vi "open_MainWindow_dyn.vi"(8 "error in (no error)":errorcluster) -> (0 "error out":errorcluster)   [LabVIEW 2015]
doc: "opens the main window dynamically"
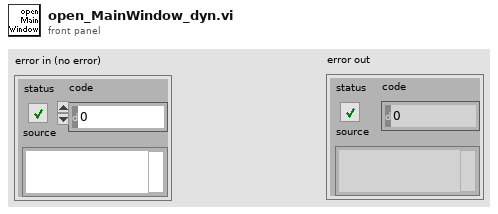
[diagram p1: front panel]
types:
  T1 = enum32{"Invalid", "Standard", "Closed", "Hidden", "Minimized", "Maximized"}
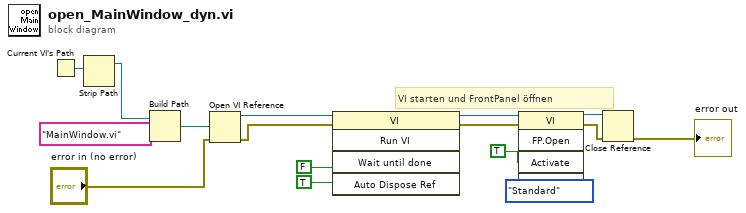
[diagram p0: block diagram]
diagram:
  # "VI starten und FrontPanel öffnen"
  n1 = Current VI's Path() -> (path=w2:path)
  n2 = Strip Path(path=w2) -> (stripped path=w1:path)  [unwired: 1 out]
  n3 = Build Path(base path=w1, name or relative path="MainWindow.vi") -> (appended path=w8:path)
  n4 = Open VI Reference(vi path=w8, error in (no error)="error in (no error)") -> (vi reference=w4:refnum<vi>, error out=w3:errorcluster)  [unwired: 4 in]
  n5 = invoke class="VI" method="Run VI"(reference=w4, error in=w3, "Wait until done"=FALSE, "Auto Dispose Ref"=TRUE) -> (reference out=w14:refnum<vi>, error out=w13:errorcluster)  [unwired: 1 in, 3 out]
  n6 = invoke class="VI" method="FP.Open"(reference=w14, error in=w13, "Activate"=TRUE, "State"=T1."Standard") -> (reference out=w10:refnum<vi>, error out=w9:errorcluster)  [unwired: 1 in, 3 out]
  n7 = Close Reference(reference=w10, error in (no error)=w9) -> (error out=→"error out":errorcluster)
